vi "strings to line.vi"(11 "strings":string[](array[string])) -> (3 "line":T1)   [LabVIEW 2013, in "EthernetIP editor node.lvclass"]
uses:
  EthernetIP editor node.lvclass
  table line.ctl
  <vilib>/NI/TBM Modules/Ethernet IP/channel/EthernetIP Channel.lvclass
  <vilib>/NI/Tag Bus/tag/Data Type.ctl
  <vilib>/NI/TBM Modules/Ethernet IP/configuration/assembly type.ctl
  <vilib>/NI/Tag Bus/tag/tag descriptor.lvclass
  <vilib>/NI/TBM Modules/Ethernet IP/configuration/EthernetIP configuration.lvclass
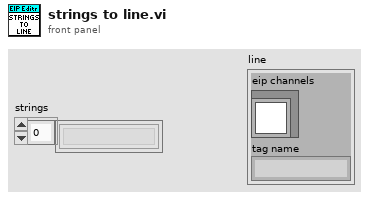
[diagram p1: front panel]
types:
  T1 = typedef "EthernetIP editor node.lvclass/table line.ctl" = cluster{"eip channels":refnum<class "EthernetIP Channel.lvclass">, "tag name":string}
  T2 = typedef "EthernetIP configuration.lvclass/assembly type.ctl" = enum32{"Producing", "Consuming"}
  T3 = typedef "tag bus.lvlib/tag descriptor.lvclass/Data Type.ctl" = enum16{"Double", "Single", "I64", "I32", "I16", "I8", "U64", "U32", "U16", "U8", "Boolean", "String", "Array of Double", "Array of Single", "Array of I64", "Array of I32", "Array of I16", "Array of I8", "Array of U64", "Array of U32", "Array of U16", "Array of U8", "Array of Boolean", "Array of String"}
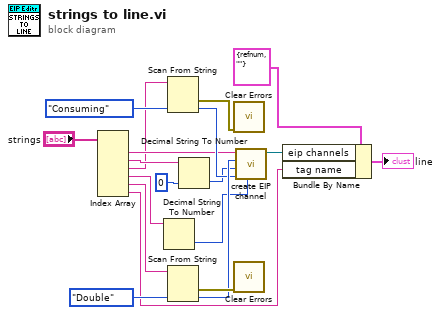
[diagram p0: block diagram]
diagram:
  n1 = Index Array(array="strings") -> (element #1=w9:string, element #2=w8:string, element #3=w5:string, element #4=w3:string, element #5=w2:string, element #6=w1:string)  [unwired: 6 in]
  n2 = Decimal String To Number(string=w3) -> (number=w4:i32)  [unwired: 2 in, 1 out]
  n3 = Scan From String(input string=w5, default 1=assembly_type."Consuming" ("Type")) -> (error out=w14:errorcluster, output 1=w10:T2)  [unwired: 3 in, 2 out]
  n4 = Scan From String(input string=w2, default 1=Data_Type."Double" ("data type")) -> (error out=w16:errorcluster, output 1=w11:T3)  [unwired: 3 in, 2 out]
  n5 = Decimal String To Number(string=w8, default (0L)=u32 0 ("Instance ID")) -> (number=w6:u32)  [unwired: 1 in, 1 out]
  n6 = call <vilib>:"Clear Errors.vi"("error in (no error)"=w14) -> ()  [unwired: 6 in, 1 out]
  n7 = call <vilib>:"Clear Errors.vi"("error in (no error)"=w16) -> ()  [unwired: 6 in, 1 out]
  n8 = call <vilib>:"create EIP channel.vi"("element"=w4, "Type"=w10, "Instance ID"=w6, "data type"=w11, "name"=w9) -> ("EthernetIP Channel out"=w12:refnum<class "EthernetIP Channel.lvclass">)  [unwired: 6 in]
  n9 = Bundle By Name(cluster=T1 {"eip channels"=refnum, "tag name"=""} ("line"), "eip channels"=w12, "tag name"=w1) -> (→"line":T1)
